vi "Write serialCommunicator.vi"(10 "serialCommunicator":refnum<class "SerialCommunicator.lvclass">, 11 "DistanceGauge in":refnum<class "DistanceGauge.lvclass">) -> (3 "DistanceGauge out":refnum<class "DistanceGauge.lvclass">)   [LabVIEW 2013, in "DistanceGauge.lvclass"]
uses:
  DistanceGauge.lvclass
  <userlib>/Common/SerialProtocols/SerialCommunicator/SerialCommunicator.lvclass
  DistanceGauge.lvclass/DistanceGauge.ctl
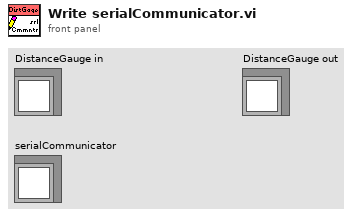
[diagram p1: front panel]
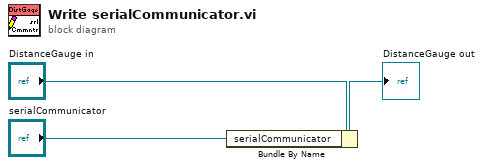
[diagram p0: block diagram]
diagram:
  n1 = Bundle By Name(cluster="DistanceGauge in", "serialCommunicator"="serialCommunicator") -> (→"DistanceGauge out":refnum<class "DistanceGauge.lvclass">)
